vi "Name Constants.vi"() -> (0 "Template Name":string="ADAS PE Template", 3 "Orignal Project Name":string="PE Template Project.lvproj", 4 "Strings to Replace w Name":string[](array[string]))   [LabVIEW 2020, in "ADAS_IO_Template_MDO.lvclass"]
uses:
  ADAS_IO_Template_MDO.lvclass
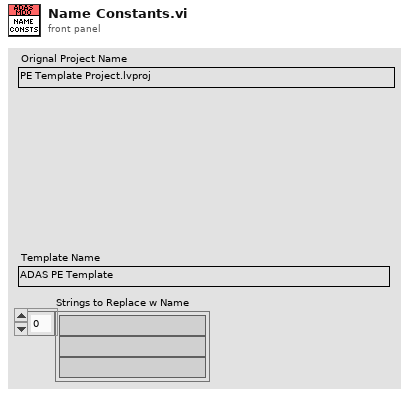
[diagram p1: front panel]
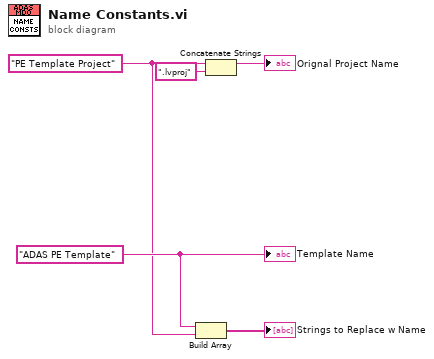
[diagram p0: block diagram]
diagram:
  w5 = "ADAS PE Template" ("name or relative path")
  w3 = "PE Template Project" ("name or relative path")
  n1 = Build Array(w5, w3) -> (→"Strings to Replace w Name":string[])
  n2 = Concatenate Strings(w3, ".lvproj" ("string")) -> (→"Orignal Project Name":string)
  "Template Name" <- w5
